vi "Kinect.vi"(10 "Mode":enum16{"Init", "Run", "End"}(ring)) -> (3 "Kinect":T1)   [LabVIEW 2011]
uses:
  <vilib>/Rock Robotics/WPI/Joystick/WPI_JoystickDeviceEnum.ctl
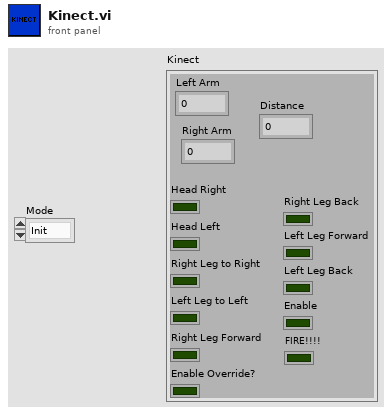
[diagram p1: front panel]
types:
  T1 = cluster{"Left Arm":dbl, "Right Arm":dbl, "Head Right":bool, "Head Left":bool, "Right Leg to Right":bool, "Left Leg to Left":bool, "Right Leg Forward":bool, "Right Leg Back":bool, "Left Leg Forward":bool, "Left Leg Back":bool, "Enable":bool, "Distance":dbl, "Enable Override?":bool, "FIRE!!!!":bool}
  T2 = typedef "WPI_JoystickDeviceEnum.ctl" = enum16{"USB 1", "USB 2", "USB 3", "USB 4", "Kinect 1", "Kinect 2"}
  T3 = typedef "WPI_JoystickDevRef.ctl" = cluster{"Device":T2}
  T4 = typedef "WPI_JoystickButtonState.ctl" = cluster{"Button 1":bool, "Button 2":bool, "Button 3":bool, "Button 4":bool, "Button 5":bool, "Button 6":bool, "Button 7":bool, "Button 8":bool, "Button 9":bool, "Button 10":bool, "Button 11":bool, "Button 12":bool}
  T5 = cluster{"axis 1 (x)":dbl, "axis 2 (y)":dbl, "axis 3 (throttle)":dbl, "axis 4":dbl, "axis 5":dbl, "axis 6":dbl}
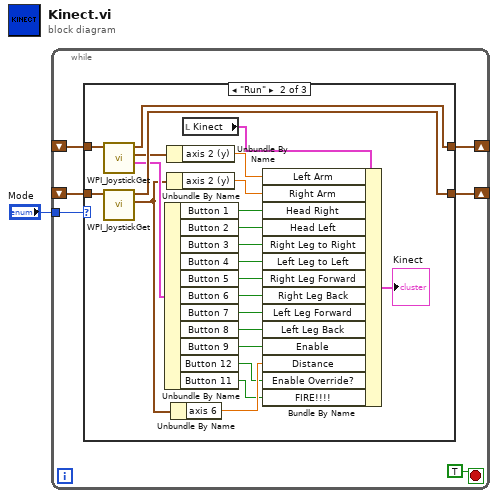
[diagram p0: block diagram]
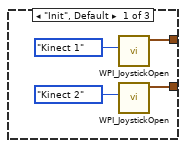
[diagram p2: hidden frame]
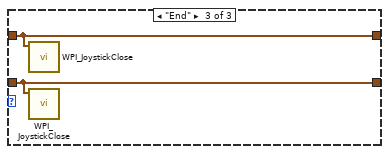
[diagram p3: hidden frame]
diagram:
  n1 = while {
    tunnel: "Mode" -> [w7]
    shift-right: [w5] -> _
    shift-left: _ -> [w3]
    shift-right: [w6] -> _
    shift-left: _ -> [w4]
    stop <- TRUE stop-if-true
    n2 = case shown="\"Run\"" w7 {
      tunnel: [w9 w32 w36] -> w6
      tunnel: [w8 w31 w35] -> w5
      tunnel: w4 -> [_ w34 w36]
      tunnel: w3 -> [_ w33 w35]
      frame "Init", Default {
        n3 = call <vilib>:"WPI_JoystickOpen.vi"("JoystickDevice"=WPI_JoystickDeviceEnum."Kinect 1") -> ("JoystickDevRef"=w9:T3)  [unwired: 10 in]
        n4 = call <vilib>:"WPI_JoystickOpen.vi"("JoystickDevice"=WPI_JoystickDeviceEnum."Kinect 2") -> ("JoystickDevRef"=w8:T3)  [unwired: 10 in]
      }
      frame "Run" {
        n5 = call <vilib>:"WPI_JoystickGet.vi"("JoystickDevRef"=w34) -> ("Buttons"=w26:T4, "Axes"=w30:T5, "JoystickDevRef"=w32:T3)  [unwired: 4 in]
        n6 = call <vilib>:"WPI_JoystickGet.vi"("JoystickDevRef"=w33) -> ("Axes"=w15:T5, "JoystickDevRef"=w31:T3)  [unwired: 4 in, 1 out]
        n7 = Unbundle By Name(w26) -> ("Button 1"=w25:bool, "Button 2"=w24:bool, "Button 3"=w23:bool, "Button 4"=w22:bool, "Button 5"=w21:bool, "Button 6"=w20:bool, "Button 7"=w19:bool, "Button 8"=w18:bool, "Button 9"=w17:bool, "Button 12"=w12:bool, "Button 11"=w13:bool)
        n8 = Unbundle By Name(w30) -> ("axis 2 (y)"=w28:dbl)
        n9 = Unbundle By Name(w15) -> ("axis 2 (y)"=w27:dbl)
        n10 = Unbundle By Name(w15) -> ("axis 6"=w14:dbl)
        n11 = local read "Kinect"() -> (w29:T1)
        n12 = Bundle By Name(cluster=w29, "Left Arm"=w28, "Right Arm"=w27, "Head Right"=w25, "Head Left"=w24, "Right Leg to Right"=w23, "Left Leg to Left"=w22, "Right Leg Forward"=w21, "Right Leg Back"=w20, "Left Leg Forward"=w19, "Left Leg Back"=w18, "Enable"=w17, "Distance"=w14, "Enable Override?"=w12, "FIRE!!!!"=w13) -> (→"Kinect":T1)
      }
      frame "End" {
        n13 = call <vilib>:"WPI_JoystickClose.vi"("JoystickDevRef"=w36) -> ()  [unwired: 11 in]
        n14 = call <vilib>:"WPI_JoystickClose.vi"("JoystickDevRef"=w35) -> ()  [unwired: 11 in]
      }
    }
  }
